vi "tdo -- do the thing -- V1.vi"(0 "Actual input file path IN":path, 1 "length":dbl, 3 "tdms file IN":refnum<k34>, 4 "Freq. threshold":dbl=30000.0 format="%#_3p", 5 "Power spctr. threshold":dbl=0.0001 format="%.2p", 6 "# of threads":i32=4, 7 "1st channel length":u64=433333, 8 "window type":enum16{"Hanning", "Box", "Blackman"}(ring), 9 "fit width":i32=9 min=3, 10 "detection method":T2(ring), 11 "step?":i64) -> (14 "Actual input file path OUT":path, 15 "amp OUT":dbl[](array[numeric]), 16 "freq OUT":dbl[](array[numeric]), 17 "tdms file OUT":refnum<k34>, 18 "time OUT":dbl[](array[numeric]), 19 "Progress":dbl(slide)=1.004382311063316 scale=0.0..1.0)   [LabVIEW 2021]
uses:
  tdo -- new/Data window.ctl
  <vilib>/Analysis/4window.llb/Hanning Window (DBL).vi
  <vilib>/Analysis/4window.llb/Blackman Window (DBL).vi
  <vilib>/Analysis/4window.llb/AllCosWindow (DBL).vi
  <vilib>/measure/matone.llb/Extract Single Tone Information 1 Chan.vi
  <vilib>/Analysis/NI_AALPro.lvlib
  <vilib>/Analysis/NI_AAL_SigProc.lvlib
  <vilib>/measure/NI_MAPro.lvlib
panel:
  in  "cignal channel":T1={"Start"=0, "Length"=500000, "Channel numbers"=[0], "Channel name"="syg", "Group name"="p"}
  # "OR"
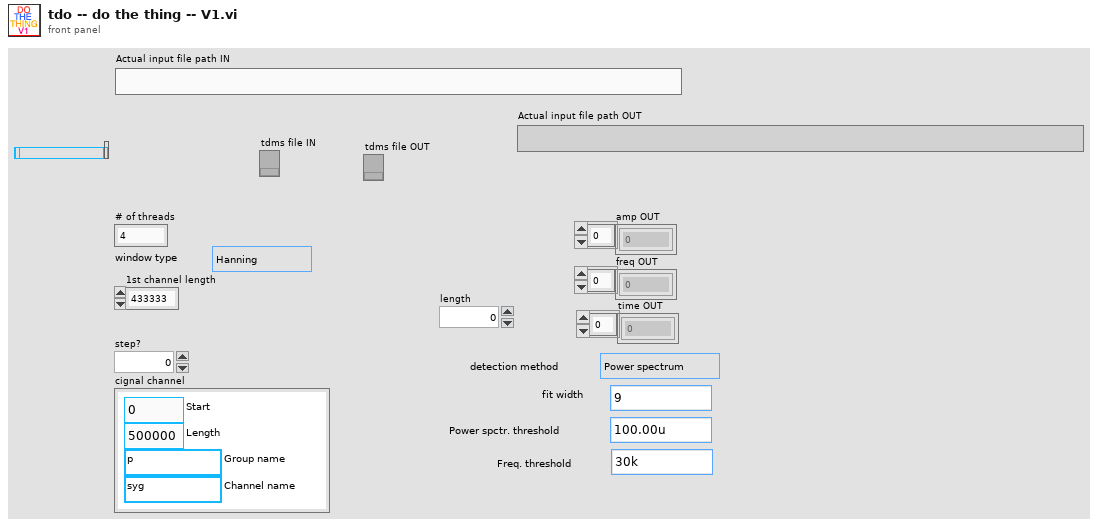
[diagram p1: front panel]
types:
  T1 = typedef "Data window.ctl" = cluster{"Start":i64, "Length":i64, "Channel numbers":i64[], "Channel name":string, "Group name":string}
  T2 = enum16{"Power spectrum", "Tone detection", "Peak-to-peak fit"}
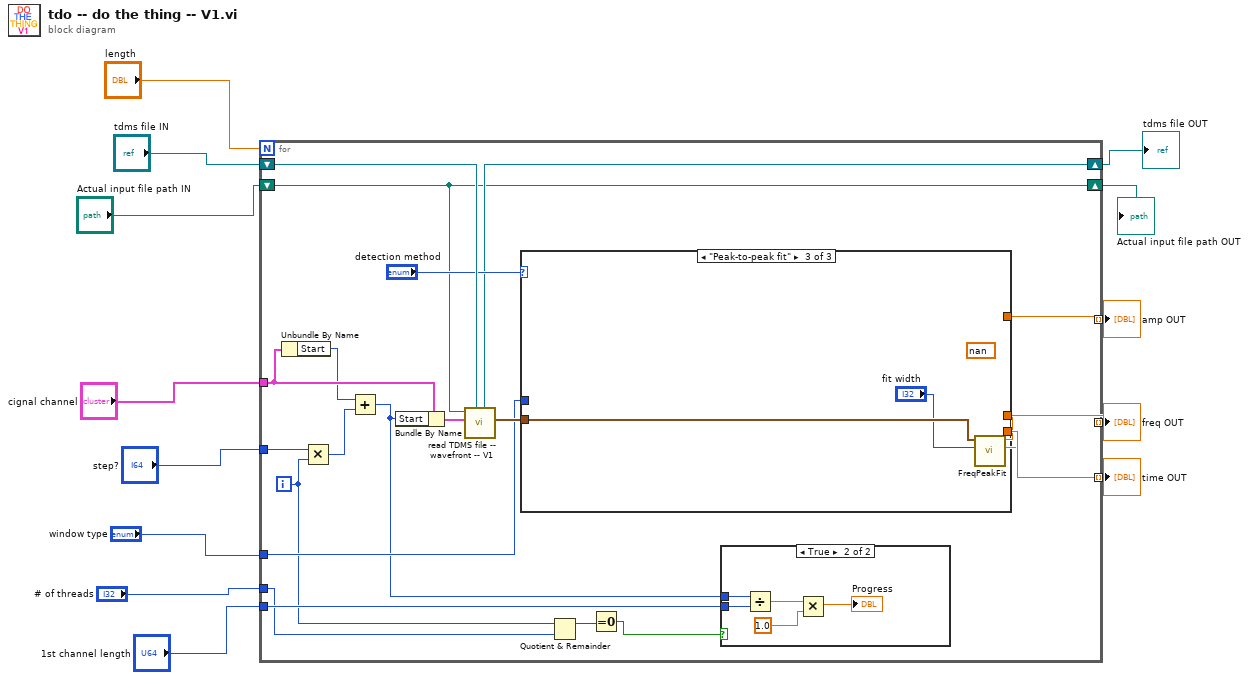
[diagram p0: block diagram]
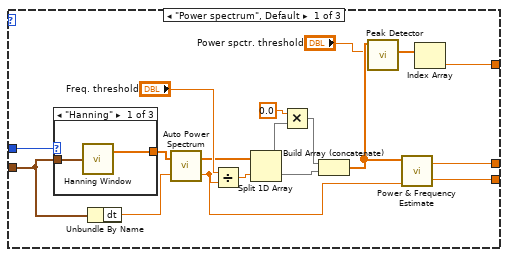
[diagram p3: hidden frame]
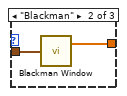
[diagram p4: hidden frame]
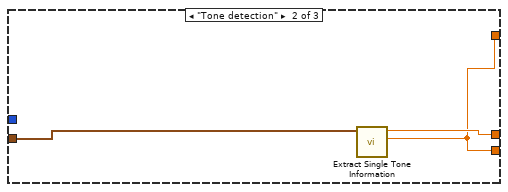
[diagram p6: hidden frame]
diagram:
  n1 = for {
    N: "length" -> [_]
    tunnel: [w31] -> w12 mode=indexing
    tunnel: [w33] -> w11 mode=indexing
    tunnel: [w32] -> w13 mode=indexing
    tunnel: "step?" -> [w28]
    tunnel: "1st channel length" -> [w30]
    tunnel: "cignal channel" -> [w15]
    tunnel: "window type" -> [w26]
    tunnel: "# of threads" -> [w19]
    shift-right: [w17] -> w2
    shift-left: "tdms file IN" -> [w20]
    shift-right: [w16] -> w3
    shift-left: "Actual input file path IN" -> [w16]
    i -> [w23]
    n2 = Unbundle By Name(w15) -> ("Start"=w14:i64)
    n3 = Multiply(x=w28, y=w23) -> (x*y=w24:i64)
    n4 = Add(x=w14, y=w24) -> (x+y=w25:i64)
    n5 = Bundle By Name(cluster=w15, "Start"=w25) -> (w27:T1)
    n6 = call "read TDMS file -- wavefront -- V1.vi"("tdms file in"=w20, "Data window"=w27, "Input file path"=w16) -> ("Data out"=w29:waveform(dbl), "tdms file out"=w17:refnum<k34>)  [unwired: 5 in, 2 out]
    n7 = case shown="\"Peak-to-peak fit\"" "detection method" {
      tunnel: [w55 w62 w65] -> w33
      tunnel: [w42 w62 w65] -> w32
      tunnel: w29 -> [w54 w63 w68]
      tunnel: [w44 w64 w67] -> w31
      tunnel: w26 -> [w45 _ _]
      frame "Power spectrum", Default {
        n8 = case shown="\"Hanning\"" w45 {
          tunnel: [w58 w60 w61] -> w56
          tunnel: w54 -> [w57 w59 w61]
          frame "Hanning" {
            n9 = call-poly <vilib>:"Hanning Window.vi"("X"=w57) -> ("Windowed X"=w58:dbl[])  [unwired: 1 out]
          }
          frame "Blackman" {
            n10 = call-poly <vilib>:"Blackman Window.vi"("X"=w59) -> ("Windowed X"=w60:dbl[])  [unwired: 1 out]
          }
          frame "Box" {
          }
        }
        n11 = Unbundle By Name(w54) -> ("dt"=w53:dbl)
        n12 = call <vilib>:"Auto Power Spectrum.vi"("dt"=w53, "Signal (V)"=w56) -> ("df"=w43:dbl, "Power Spectrum (V^2 rms)"=w51:dbl[])
        n13 = Divide(x="Freq. threshold", y=w43) -> (x/y=w50:dbl)
        n14 = Split 1D Array(array=w51, index=w50) -> (first subarray=w47:dbl[], second subarray=w49:dbl[])
        n15 = Multiply(x=0.0 ("element"), y=w47) -> (x*y=w46:dbl[])
        n16 = Build Array (concatenate)(w46, w49) -> (w41:dbl[])
        n17 = call <vilib>:"Peak Detector.vi"("threshold"="Power spctr. threshold", "X"=w41) -> ("Amplitudes"=w39:dbl[])  [unwired: 5 in, 4 out]
        n18 = call <vilib>:"Power & Frequency Estimate.vi"("df"=w43, "Power Spectrum (V^2 rms)"=w41) -> ("est power peak"=w55:dbl, "est frequency peak"=w44:dbl)  [unwired: 3 in, 1 out]
        n19 = Index Array(array=w39) -> (element=w42:dbl)  [unwired: 1 in]
      }
      frame "Tone detection" {
        n20 = call-poly <vilib>:"Extract Single Tone Information.vi"("time signal in"=w63) -> ("detected amplitude"=w62:dbl, "detected frequency"=w64:dbl)  [unwired: 3 in, 6 out]
      }
      frame "Peak-to-peak fit" {
        (unwired) nan
        n21 = call "FreqPeakFit.vi"("Peak fit width"="fit width", "Waveform"=w68) -> ("Amplitude"=w65:dbl, "PeakFreqOut"=w67:dbl)  [unwired: 1 in, 5 out]
      }
    }
    n22 = Quotient & Remainder(x=w23, y=w19) -> (x-y*floor(x/y)=w22:i32)  [unwired: 1 out]
    n23 = Equal To 0?(x=w22) -> (x = 0?=w21:bool)
    n24 = case shown="True" w21 {
      tunnel: w30 -> [_ w38]
      tunnel: w25 -> [_ w35]
      frame False {
      }
      frame True {
        n25 = Divide(x=w35, y=w38) -> (x/y=w37:dbl)
        n26 = Multiply(x=w37, y=1.0) -> (x*y=→"Progress":dbl)
      }
    }
  }
  "amp OUT" <- w13
  "freq OUT" <- w12
  "time OUT" <- w11
  "Actual input file path OUT" <- w3
  "tdms file OUT" <- w2
